vi "GetFileList.vi"(5 "error in (no error)":errorcluster) -> (14 "filenames":string[](array[string]), 19 "error out":errorcluster)   [LabVIEW 2014, in "IndoorData.lvclass"]
uses:
  IndoorData.lvclass
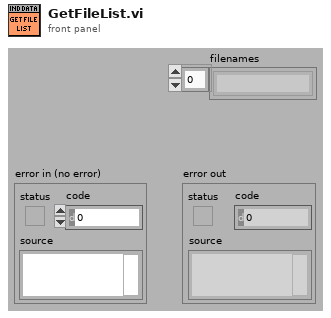
[diagram p1: front panel]
types:
  T1 = typedef "IndoorData.lvclass/ObjectAttributes.ctl" = cluster{"DebugData":T2, "Actual":T3, "BufferedReadings":T4, "AVGReadings":T4, "DataFolder":path}
  T2 = typedef "IndoorData.lvclass/DebugData.ctl" = cluster{"Rev":string, "Location":string, "LoopIdx":i32, "PiCoreTemp":dbl, "Error":errorcluster}
  T3 = typedef "IndoorData.lvclass/ActualValues.ctl" = cluster{"Time":dbl, "Temp":dbl, "RH":dbl}
  T4 = typedef "IndoorData.lvclass/BufferedReadings.ctl" = cluster{"Time":dbl[], "Temp":dbl[], "RH":dbl[]}
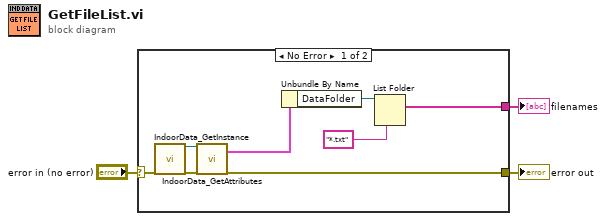
[diagram p0: block diagram]
diagram:
  n1 = case shown="No Error" "error in (no error)" {
    selector: "error in (no error)" -> [w9 w12]
    tunnel: [w11 w12] -> w2
    tunnel: [w4 _] -> w1
    frame No Error {
      n2 = call "IndoorData_GetInstance.vi"("error in (no error)"=w9) -> ("reference out"=w10:refnum<class "IndoorData.lvclass">, "error out"=w8:errorcluster)  [unwired: 14 in, 3 out]
      n3 = call "IndoorData_GetAttributes.vi"("reference in"=w10, "error in (no error)"=w8) -> ("Data"=w5:T1, "error out"=w11:errorcluster)  [unwired: 14 in, 2 out]
      n4 = Unbundle By Name(w5) -> ("DataFolder"=w7:path)
      n5 = List Folder(path=w7, pattern="*.txt") -> (filenames=w4:string[])  [unwired: 2 in, 3 out]
    }
    frame Error {
    }
  }
  "error out" <- w2
  "filenames" <- w1
